vi "Constants.vi"() -> ()   [LabVIEW 2017, in "PXImc Shared.lvlib"]
doc: "Use this Global VI to access the GUIDs assigned to the page resources of the Custom Device."
uses:
  PXImc Shared.lvlib
  Channel.ctl
panel:
  in  "Tab Control":enum32{"GUIDS", "Constants", "Properties"}(tab)=enum."Properties"
  in  "Custom Device Disabled":string="23168F61-B105-D978-DB9A-9F8ED3C6E22D_DISABLED"
  in  "Chan Del Prot":string="C9C36D38-F811-822C-0C95-B5EFD5033E75"
  in  "Sect Del Prot":string="297B72C6-21C2-EA0B-6E7C-23F9EC8798A9"
  in  "Custom Device":string="23168F61-B105-D978-DB9A-9F8ED3C6E22D"
  in  "Status Chans":T1[](array[typedef])=[{"Name"="Write Duration", "Units"="S", "Default"=0.0, "Description"="Duration of code execution to read the NIVS channels and write them to PXImc"}, {"Name"="Read Duration", "Units"="S", "Default"=0.0, "Description"="Duration of code execution to read the PXImc data and write it to the NIVS channels"}, {"Name"="Read Buffer Low", "Units"="", "Default"=0.0, "Description"="Number of times PXImc read buffer did not contain enough elements to read from, indicating the data had not yet arrived"}, {"Name"="Write Late Count", "Units"="", "Default"=0.0, "Description"="Number of times PXImc write failed to write any data, indicating the reader has not yet read data from previous iterations"}, {"Name"="Read Buffer Full", "Units"="", "Default"=0.0, "Description"="Number of times PXImc read buffer was full, indicating the data was stale and had to be discarded"}]
  in  "Imp_Exp Config File Path":string="Imp_Exp Config File Path"
  in  "ModName":string="ModName"
  in  "RemoteWriterID":string="RemoteWriterID"
  in  "MyWriterID":string="WriterID"
  in  "CompiledData":string="CompiledData"
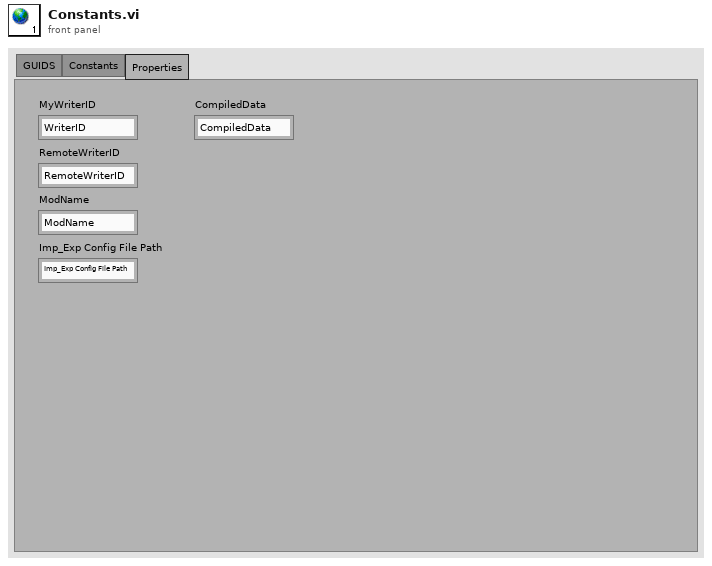
[diagram p1: front panel]
types:
  T1 = typedef "PXImc Shared.lvlib/Channel.ctl" = cluster{"Name":string, "Units":string, "Default":dbl, "Description":string}
diagram:
